vi "Host DDS Generation Calculate FPGA Parameters.vi"(5 "Accumulator Size (bit)":i32=32, 6 "Amplitude Scaling Parameters":T1={"Full Scale (V) "=10.0, "Full Scale (binary)"=32768.0}, 7 "Loop Rate (Hz)":dbl, 9 "Signal Amplitude (V)":dbl=5.0, 10 "Phase Shift (Deg)":dbl, 11 "DDS Signal Frequency (Hz)":dbl=20000.0) -> (0 "Phase Shift Cos":u32, 1 "AO Amplitude":u16, 2 "Phase Shift Sin":u32, 3 "Accumulator Increment":u32, 4 "Scaling Ratio":dbl)   [LabVIEW 2009]
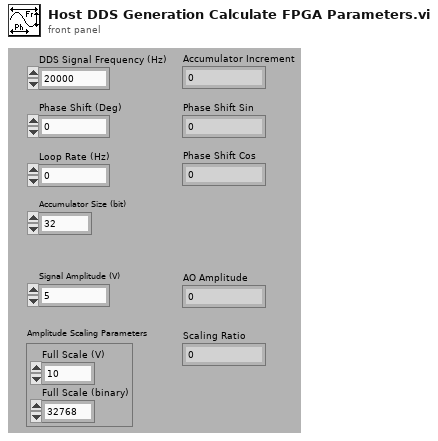
[diagram p1: front panel]
types:
  T1 = cluster{"Full Scale (V) ":dbl, "Full Scale (binary)":dbl}
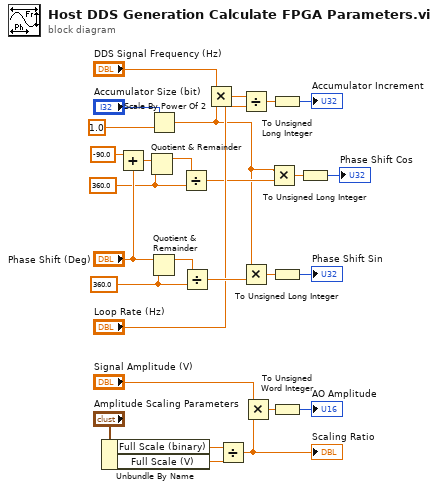
[diagram p0: block diagram]
diagram:
  w2 = 360.0 ("y")
  w10 = 360.0 ("y")
  n1 = Unbundle By Name("Amplitude Scaling Parameters") -> ("Full Scale (binary)"=w16:dbl, "Full Scale (V)"=w15:dbl)
  n2 = Add(x=-90.0, y="Phase Shift (Deg)") -> (x+y=w3:dbl)
  n3 = Quotient & Remainder(x=w3, y=w2) -> (x-y*floor(x/y)=w1:dbl)  [unwired: 1 out]
  n4 = Scale By Power Of 2(n="Accumulator Size (bit)", x=1.0) -> (x*2^n=w4:dbl)
  n5 = Quotient & Remainder(x="Phase Shift (Deg)", y=w10) -> (x-y*floor(x/y)=w11:dbl)  [unwired: 1 out]
  n6 = Divide(x=w1, y=w2) -> (x/y=w7:dbl)
  n7 = Divide(x=w11, y=w10) -> (x/y=w24:dbl)
  n8 = Multiply(x="DDS Signal Frequency (Hz)", y=w4) -> (x*y=w23:dbl)
  n9 = Divide(x=w16, y=w15) -> (x/y=w14:dbl)
  "Scaling Ratio" <- w14
  n10 = Divide(x=w23, y="Loop Rate (Hz)") -> (x/y=w27:dbl)
  n11 = Multiply(x=w4, y=w24) -> (x*y=w19:dbl)
  n12 = Multiply(x="Signal Amplitude (V)", y=w14) -> (x*y=w21:dbl)
  n13 = Multiply(x=w4, y=w7) -> (x*y=w6:dbl)
  n14 = To Unsigned Long Integer(number=w27) -> (unsigned 32bit integer=→"Accumulator Increment":u32)
  n15 = To Unsigned Long Integer(number=w19) -> (unsigned 32bit integer=→"Phase Shift Sin":u32)
  n16 = To Unsigned Word Integer(number=w21) -> (unsigned 16bit integer=→"AO Amplitude":u16)
  n17 = To Unsigned Long Integer(number=w6) -> (unsigned 32bit integer=→"Phase Shift Cos":u32)
